vi "K8055_sim.vi"(1 "Hardware":bool, 2 "Fan Speed":u8(knob) scale=0.0..255.0) -> (0 "Read temp":dbl)   [LabVIEW 2024]
uses:
  Global 1.vi
  K8055D.dll
panel:
  out "Numeric":dbl
  in  "Knob 2":dbl(knob) scale=0.0..255.0
  in  "Card":dbl
  out "Boolean 12":bool
  out "Boolean 11":bool
  out "Boolean 10":bool
  out "Boolean 13":bool
  out "Boolean 9":bool
  in  "Boolean 8":bool
  in  "Boolean 7":bool
  in  "Boolean 6":bool
  in  "Boolean 5":bool
  in  "Boolean 4":bool
  in  "Boolean 3":bool
  in  "Boolean 2":bool
  in  "Boolean 1":bool
  # "Simulation"
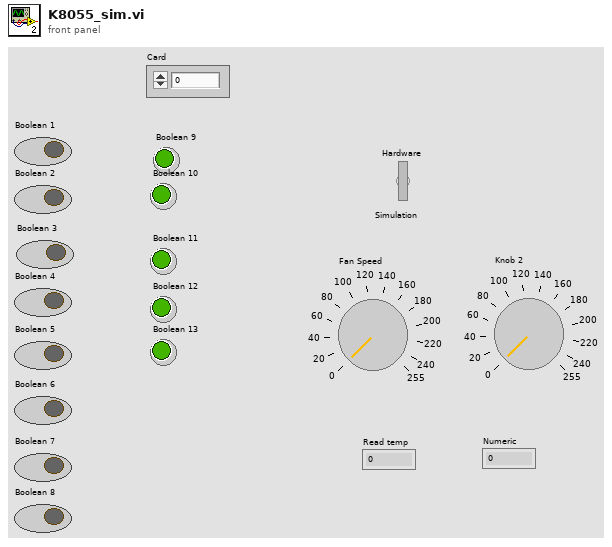
[diagram p1: front panel]
types:
  T1 = cluster{"Boolean array[0]":bool, "Boolean array[1]":bool, "Boolean array[2]":bool, "Boolean array[3]":bool, "Boolean array[4]":bool, "Boolean array[5]":bool, "Boolean array[6]":bool, "Boolean array[7]":bool, "Boolean array[8]":bool}
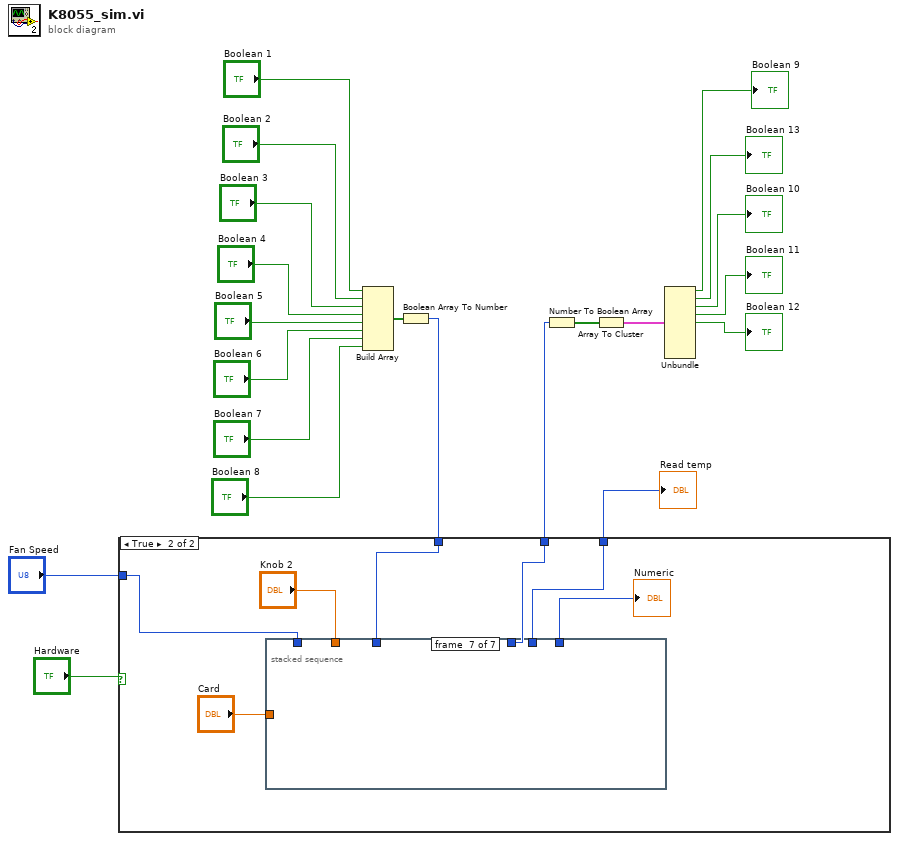
[diagram p0: block diagram]
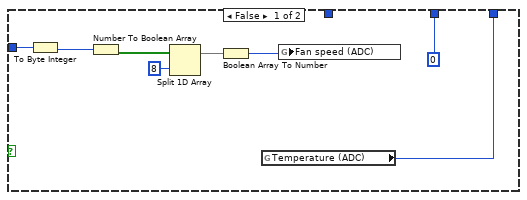
[diagram p2: hidden frame]
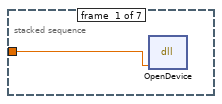
[diagram p3: hidden frame]
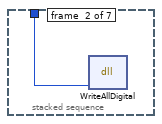
[diagram p4: hidden frame]
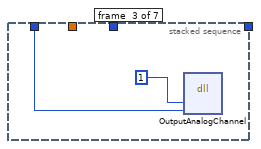
[diagram p5: hidden frame]
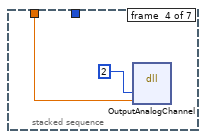
[diagram p6: hidden frame]
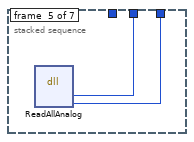
[diagram p7: hidden frame]
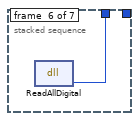
[diagram p8: hidden frame]
diagram:
  n1 = Build Array("Boolean 1", "Boolean 2", "Boolean 3", "Boolean 4", "Boolean 5", "Boolean 6", "Boolean 7", "Boolean 8") -> (w11:bool[])
  n2 = Boolean Array To Number(Boolean array=w11) -> (number=w10:u32)
  n3 = case shown="True" "Hardware" {
    tunnel: [w29 w31] -> w9
    tunnel: "Fan Speed" -> [w28 w33]
    tunnel: w10 -> [_ w36]
    tunnel: [0 w30] -> w8
    frame False {
      n4 = To Byte Integer(number=w28) -> (8bit integer=w27:i8)
      n5 = Number To Boolean Array(number=w27) -> (Boolean array=w26:bool[])
      n6 = Split 1D Array(array=w26, index=8) -> (first subarray=w23:bool[])  [unwired: 1 out]
      n7 = Boolean Array To Number(Boolean array=w23) -> (number=w24:u32)
      n8 = global read "Global 1.vi" "Temperature (ADC)"() -> (w29:u8)
      n9 = global write "Global 1.vi" "Fan speed (ADC)"(w24) -> ()
    }
    frame True {
      n10 = stacked-sequence {
        tunnel: w36 -> [_ w38 _ _ _ _ _]
        tunnel: "Card" -> [w37 _ _ _ _ _ _]
        tunnel: "Knob 2" -> [_ _ _ w41 _ _ _]
        tunnel: w33 -> [_ _ w39 _ _ _ _]
        tunnel: [_ _ _ _ w44 _ _] -> w31
        tunnel: [_ _ _ _ w43 _ _] -> w32
        tunnel: [_ _ _ _ _ w45 _] -> w30
        frame #0 {
          n11 = dll-call lib="E:/Auston Applied Instrumentation/K8055D.dll" fn="OpenDevice"("arg1"=w37) -> ()  [unwired: 5 in, 2 out]
        }
        frame #1 {
          n12 = dll-call lib="E:/Auston Applied Instrumentation/K8055D.dll" fn="WriteAllDigital"("arg1"=w38) -> ()  [unwired: 5 in, 2 out]
        }
        frame #2 {
          n13 = dll-call lib="E:/Auston Applied Instrumentation/K8055D.dll" fn="OutputAnalogChannel"(1, "arg2"=w39) -> ()  [unwired: 6 in, 2 out]
        }
        frame #3 {
          n14 = dll-call lib="E:/Auston Applied Instrumentation/K8055D.dll" fn="OutputAnalogChannel"(2, "arg2"=w41) -> ()  [unwired: 6 in, 2 out]
        }
        frame #4 {
          n15 = dll-call lib="E:/Auston Applied Instrumentation/K8055D.dll" fn="ReadAllAnalog"() -> ("arg1"=w44:i32, "arg2"=w43:i32)  [unwired: 6 in, 2 out]
        }
        frame #5 {
          n16 = dll-call lib="E:/Auston Applied Instrumentation/K8055D.dll" fn="ReadAllDigital"() -> ("return type"=w45:i32)  [unwired: 3 in, 2 out]
        }
        frame #6 {
        }
      }
      "Numeric" <- w32
    }
  }
  "Read temp" <- w9
  n17 = Number To Boolean Array(number=w8) -> (Boolean array=w7:bool[])
  n18 = Array To Cluster(array=w7) -> (cluster=w6:T1)
  n19 = Unbundle(w6) -> ("Boolean array[0]"=→"Boolean 9":bool, "Boolean array[1]"=→"Boolean 13":bool, "Boolean array[2]"=→"Boolean 10":bool, "Boolean array[3]"=→"Boolean 11":bool, "Boolean array[4]"=→"Boolean 12":bool)  [unwired: 4 out]
